vi "FPGA Addon System Definition API Example.vi"() -> ()   [LabVIEW 2018]
uses:
  NationalInstruments.VeriStand.Internal
  NationalInstruments.VeriStand.SystemDefinitionAPI
  FPGA System Definition API.lvlib
panel:
  out "Sysdef Path":path=path "C:/Users/Public/Documents/National Instruments/NI VeriStand 2015/Projects/DynamicallyCreatedProject/DynamicallyCreatedProject.nivssdf"
  in  "error in (no error)":errorcluster
  out "error out":errorcluster
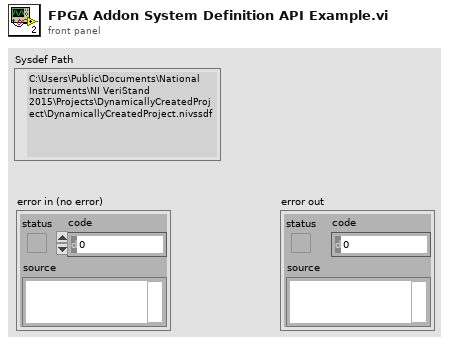
[diagram p1: front panel]
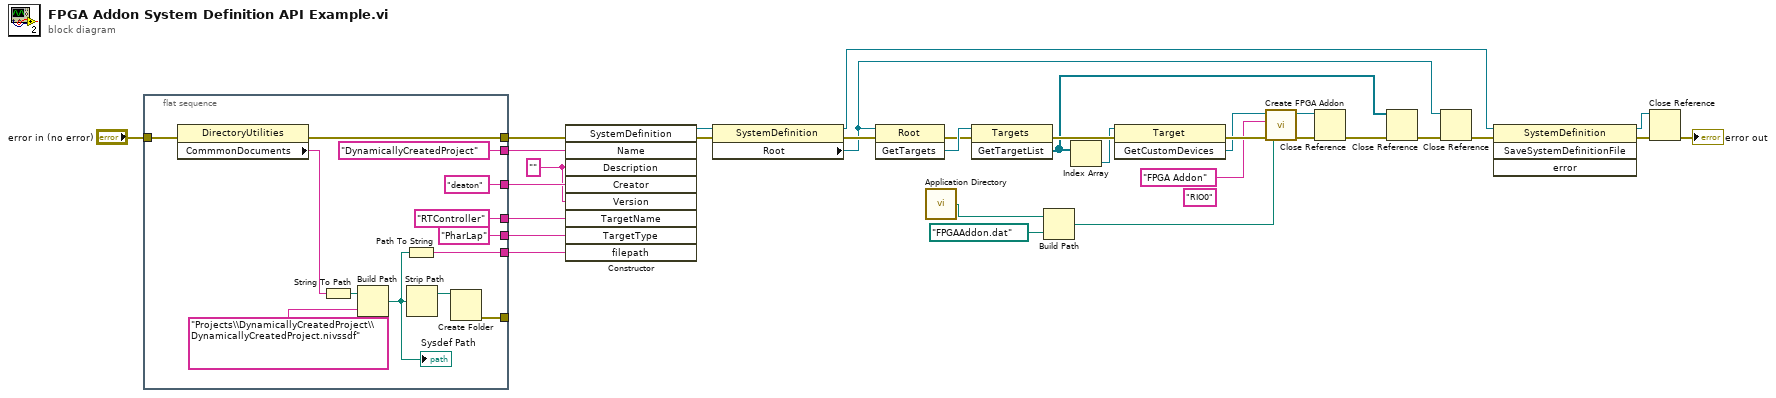
[diagram p0: block diagram]
diagram:
  (unwired) "RIO0" ("RIO Device")
  w29 = "" ("Description")
  n1 = flat-sequence {
    tunnel: ["DynamicallyCreatedProject" ("Name")] -> w32
    tunnel: ["deaton" ("Creator")] -> w31
    tunnel: ["PharLap" ("TargetType")] -> w30
    tunnel: [w42] -> w28
    tunnel: ["RTController" ("TargetName")] -> w22
    tunnel: "error in (no error)" -> [w35]
    tunnel: [w34] -> w8
    tunnel: [w33] -> _
    frame #0 {
      n2 = property class="DirectoryUtilities"(error in=w35) -> (error out=w34:errorcluster, "CommmonDocuments"=w39:string)  [unwired: 1 in, 1 out]
      n3 = String To Path(string=w39) -> (path=w38:path)
      n4 = Build Path(base path=w38, name or relative path="Projects\\DynamicallyCreatedProject\\DynamicallyCreatedProject.nivssdf") -> (appended path=w36:path)
      "Sysdef Path" <- w36
      n5 = Path To String(path=w36) -> (string=w42:string)
      n6 = Strip Path(path=w36) -> (stripped path=w40:path)  [unwired: 1 out]
      n7 = Create Folder(path (use dialog)=w40) -> (error out=w33:errorcluster)  [unwired: 2 in, 2 out]
    }
  }
  n8 = constructor class="SystemDefinition"(error in=w8, "Name"=w32, "Description"=w29, "Creator"=w31, "Version"=w29, "TargetName"=w22, "TargetType"=w30, "filepath"=w28) -> (reference out=w24:refnum<k24>, error out=w26:errorcluster)  [unwired: 2 in, 8 out]
  n9 = property class="SystemDefinition"(reference=w24, error in=w26) -> (reference out=w12:refnum<k24>, error out=w25:errorcluster, "Root"=w11:refnum<k24>)
  n10 = invoke class="Root" method="GetTargets"(reference=w11, error in=w25) -> (error out=w23:errorcluster, "GetTargets"=w27:refnum<k24>)  [unwired: 1 in, 1 out]
  n11 = call <vilib>:"Application Directory.vi"() -> ("Application Directory"=w1:path)
  n12 = invoke class="Targets" method="GetTargetList"(reference=w27, error in=w23) -> (error out=w21:errorcluster, "GetTargetList"=w10:refnum<k24>[])  [unwired: 1 in, 1 out]
  n13 = Build Path(base path=w1, name or relative path=path "FPGAAddon.dat" ("Path (.dat)")) -> (appended path=w2:path)
  n14 = Index Array(array=w10) -> (element=w20:refnum<k24>)  [unwired: 1 in]
  n15 = invoke class="Target" method="GetCustomDevices"(reference=w20, error in=w21) -> (error out=w14:errorcluster, "GetCustomDevices"=w5:refnum<k24>)  [unwired: 1 in, 1 out]
  n16 = call "Create FPGA Addon.vi"("Configuration (.dat)"=w2, "error in (no error)"=w14, "Name"="FPGA Addon", "Custom Devices Ref"=w5) -> ("error out"=w7:errorcluster, "Custom Devices Ref"=w13:refnum<k24>)  [unwired: 6 in]
  n17 = Close Reference(reference=w13, error in (no error)=w7) -> (error out=w6:errorcluster)
  n18 = Close Reference(reference=w10, error in (no error)=w6) -> (error out=w18:errorcluster)
  n19 = Close Reference(reference=w11, error in (no error)=w18) -> (error out=w19:errorcluster)
  n20 = invoke class="SystemDefinition" method="SaveSystemDefinitionFile"(reference=w12, error in=w19) -> (reference out=w17:refnum<k24>, error out=w15:errorcluster)  [unwired: 2 in, 2 out]
  n21 = Close Reference(reference=w17, error in (no error)=w15) -> (error out=→"error out":errorcluster)
